vi "Configure Continuous Acquisition.vi"(8 "error in (no error)":errorcluster, 9 "Auto Trigger (T)":bool=TRUE, 10 "Enable Continuous Acquisition(T: On)":bool=TRUE, 11 "VISA resource name":refnum<visa-resource-name>) -> (0 "error out":errorcluster, 3 "VISA resource name out":refnum<visa-resource-name>)   [LabVIEW 2021, in "Siglent SDS 1000 2000 Series.lvlib"]
doc: "Configures the instrument to run continuously or to stop after a single configured acquisition.\n\nNote:\n(1) This setting does not occur until the <B>Initiate</B> or <B>Read Waveform</B> VI is called.\n(2) Performing an Autosetup, will put the instrument in continuous acquisition mode."
uses:
  <instrlib>/Siglent SDS 1000 2000 Series/Siglent SDS 1000 2000 Series.lvlib
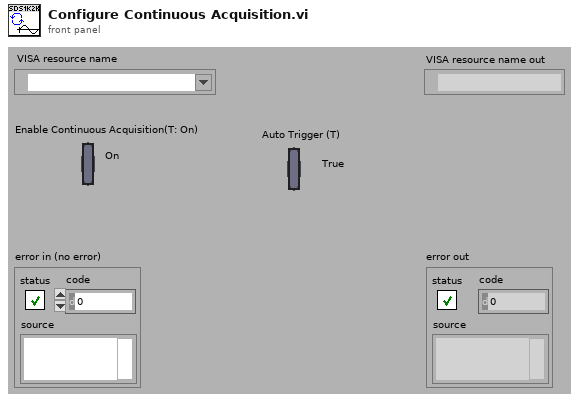
[diagram p1: front panel]
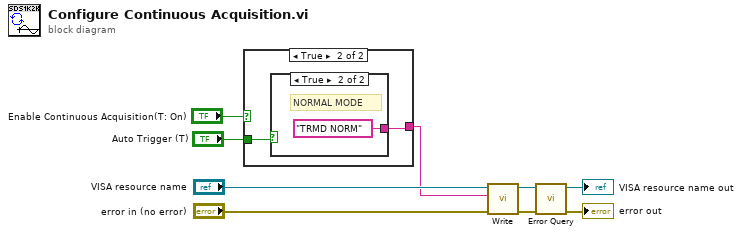
[diagram p0: block diagram]
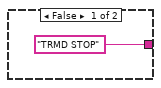
[diagram p2: hidden frame]
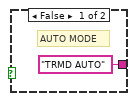
[diagram p3: hidden frame]
diagram:
  n1 = case shown="True" "Enable Continuous Acquisition(T: On)" {
    tunnel: ["TRMD STOP" w11] -> w2
    tunnel: "Auto Trigger (T)" -> [_ w12]
    frame False {
    }
    frame True {
      n2 = case shown="True" w12 {
        tunnel: ["TRMD AUTO" "TRMD NORM"] -> w11
        frame False {
          # "AUTO MODE"
        }
        frame True {
          # "NORMAL MODE"
        }
      }
    }
  }
  n3 = call <instrlib>:"Write.vi"("error in (no error)"="error in (no error)", "Write Buffer"=w2, "VISA resource name"="VISA resource name") -> ("error out"=w5:errorcluster, "VISA resource name out"=w6:refnum<visa-resource-name>)  [unwired: 6 in, 1 out]
  n4 = call <instrlib>:"Error Query.vi"("error in (no error)"=w5, "VISA resource name"=w6) -> ("error out"=→"error out":errorcluster, "VISA resource name out"=→"VISA resource name out":refnum<visa-resource-name>)  [unwired: 6 in, 2 out]
